vi "Tests Basic COBS.vi"() -> ()   [LabVIEW 2015, in "LSR Transmission.lvlib"]
uses:
  LSR Transmission.lvlib
panel:
  out "Stuffed size":i32
  out "Array Sizes Out":i32
  out "Array Sizes":i32
  out "logical AND":bool
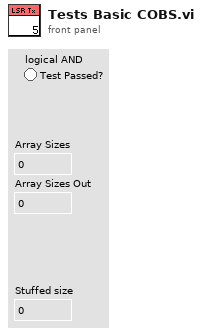
[diagram p1: front panel]
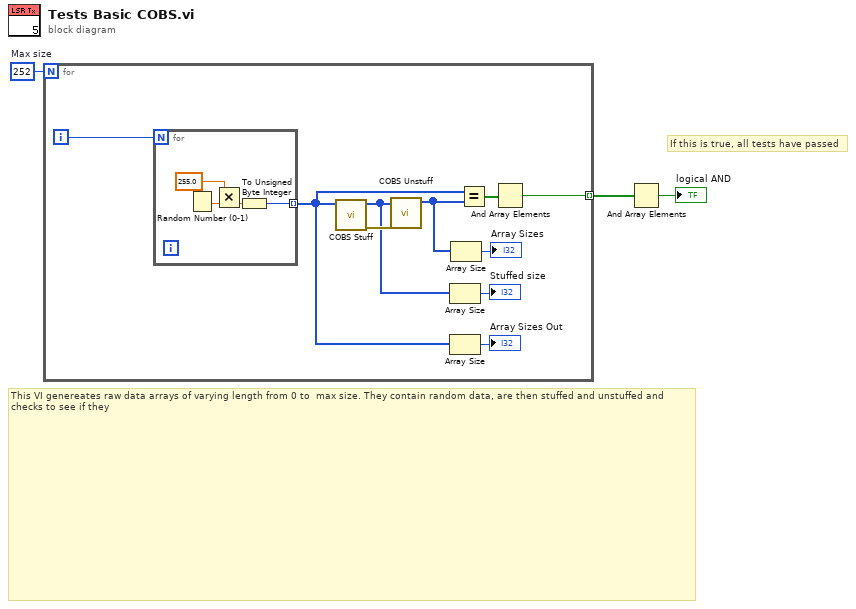
[diagram p0: block diagram]
diagram:
  w3 = 252  # Max size
  # "This VI genereates raw data arrays of varying length from 0 to  max size. They contain random data, are then stuffed and unstuffed and checks to see if they"
  # "If this is true, all tests have passed"
  n1 = for {
    N: w3 -> [_]
    tunnel: [w10] -> w2 mode=indexing
    i -> [w13]
    n2 = for {
      N: w13 -> [_]
      tunnel: [w17] -> w9 mode=indexing
      n3 = Random Number (0-1)() -> (number: 0 to 1=w14:dbl)
      n4 = Multiply(x=255.0, y=w14) -> (x*y=w15:dbl)
      n5 = To Unsigned Byte Integer(number=w15) -> (unsigned 8bit integer=w17:u8)
    }
    n6 = call "COBS Stuff.vi"("Raw Array in"=w9) -> ("error out"=w12:errorcluster, "Stuffed Array out"=w4:u8[])  [unwired: 9 in]
    n7 = call "COBS Unstuff.vi"("error in (no error)"=w12, "Stuffed data in"=w4) -> ("Unstuffed Data"=w8:u8[])  [unwired: 7 in, 2 out]
    n8 = Array Size(array=w4) -> (size(s)=→"Stuffed size":i32)
    n9 = Array Size(array=w9) -> (size(s)=→"Array Sizes Out":i32)
    n10 = Array Size(array=w8) -> (size(s)=→"Array Sizes":i32)
    n11 = Equal?(x=w9, y=w8) -> (x = y?=w11:bool[])
    n12 = And Array Elements(Boolean array=w11) -> (logical AND=w10:bool)
  }
  n13 = And Array Elements(Boolean array=w2) -> (logical AND=→"logical AND":bool)
